vi "Event Handler.vi"(0 "uService Template in":refnum<class "Father of all uServices.lvclass">, 5 "Event type":T1=enum."Message", 7 "Item Name":string, 9 "Data":variant, 11 "error in (no error)":errorcluster) -> (4 "uService Template out":refnum<class "Father of all uServices.lvclass">, 15 "error out":errorcluster)   [LabVIEW 2026, in "TALOS.lvlib" / "Father of all uServices.lvlib" / "Father of all uServices.lvclass"]
uses:
  Father of all uServices.lvclass
  Event Handler Items.ctl
  Father of all uServices.lvclass/Father of all uServices.ctl
  Ancestor/Ancestor/Ancestor.lvclass/Ancestor.ctl
  Classes/Log/Log.lvclass/Log.ctl
  <vilib>/AdvancedString/1D String Array to Delimited String (string).vi
  Support VIs/Generate Error.vi
  Classes/Log/Write.vi
  FGV/Error Memory/Get Error Description.vi
  Support VIs/Get PC name.vi
  Ancestor/Ancestor/Read ID.vi
  Support VIs/Get Class Name.vi
  Support VIs/Date n Time.vi
  FGV/Error Memory/Error Memory Core.vi
  <vilib>/AdvancedString/Delimited String to 1D String Array.vi
  <vilib>/AdvancedString/Delimited String to 1D String Array (string).vi
  Support VIs/Circus Root Path.vi
  FGV/Error Memory/Error Crt Lvl checker.vi
  FGV/Error Memory/Error Memory Core.vi/40c8088d-b597-4017-91af-faa98e00292e.vi
  FGV/Error Memory/Error Memory Core.vi/d4a3ab98-063c-4e44-b43d-fbdcfe6c2be2.vi
  Support VIs/Global Memory.vi
  <vilib>/Utility/LVClass/Get LV Class Name.vi
  Support VIs/Is in Packed Library.vi
  Support VIs/TALOS Root path.vi
  Support VIs/Read CSV worksheet.vi
  Support VIs/Global Constants.vi
  <vilib>/Utility/error.llb/General Error Handler.vi
  <vilib>/Utility/config.llb/Open Config Data.vi
  <vilib>/Utility/config.llb/Get Section Names.vi
  <vilib>/Utility/config.llb/Get Key Names.vi
  <vilib>/Utility/config.llb/Read Key.vi
  <vilib>/Utility/config.llb/Read Key (String).vi
  <vilib>/Utility/config.llb/Close Config Data.vi
  Classes/Log/Rotate.vi
  Ancestor/Ancestor/Ancestor.lvclass
  <vilib>/Comparison/Equal/Equal Functor/Equal Functor.lvclass
  TALOS.lvlib
  Classes/Log/Log.lvclass
panel:
  # "NEVER REGENERATE THE AF MESSAGE!\nIT IS MANUALLY MODIFIED"
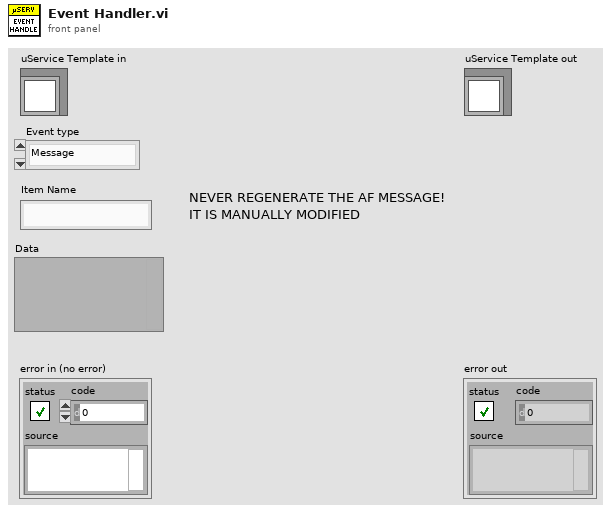
[diagram p1: front panel]
types:
  T1 = typedef "TALOS.lvlib/Father of all uServices.lvlib/Father of all uServices.lvclass/Event Handler Items.ctl" = enum16{"Button Pressed", "Message", "Ready to launch?", "Safe Mode", "Start RUN", "Stop RUN"}
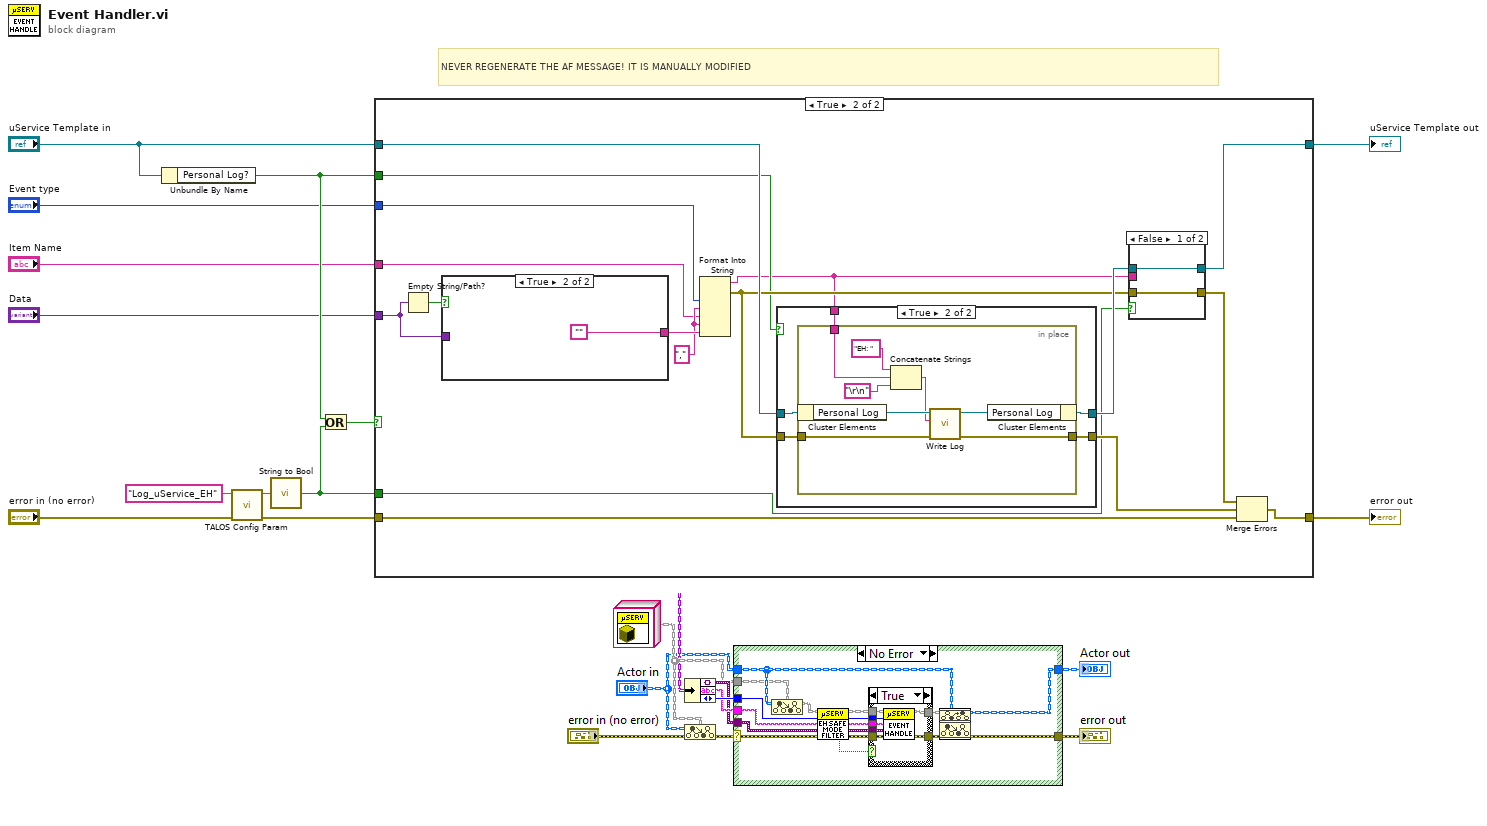
[diagram p0: block diagram]
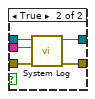
[diagram p3: hidden frame]
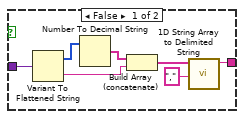
[diagram p4: hidden frame]
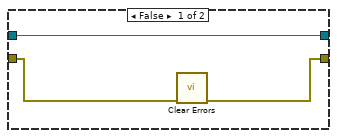
[diagram p5: hidden frame]
diagram:
  # "NEVER REGENERATE THE AF MESSAGE! IT IS MANUALLY MODIFIED"
  n1 = Unbundle By Name("uService Template in") -> ("Personal Log?"=w6:bool)
  n2 = call "TALOS Config Param.vi"("error in (no error)"="error in (no error)", "Parameter Name"="Log_uService_EH") -> ("error out"=w9:errorcluster, "Output"=w11:string)  [unwired: 8 in]
  n3 = call "String to Bool.vi"("String"=w11) -> ("Boolean"=w5:bool)
  n4 = Or(x=w6, y=w5) -> (x .or. y?=w7:bool)
  n5 = case shown="True" w7 {
    tunnel: [w14 w32] -> w13
    tunnel: [w15 w29] -> w12
    tunnel: "Item Name" -> [_ w27]
    tunnel: "Event type" -> [_ w26]
    tunnel: "uService Template in" -> [w14 w22]
    tunnel: "Data" -> [_ w25]
    tunnel: w9 -> [w15 w24]
    tunnel: w6 -> [_ w18]
    tunnel: w5 -> [_ w16]
    frame False {
    }
    frame True {
      w28 = "," ("input 2")
      n6 = Empty String/Path?(string/path=w25) -> (empty?=w31:bool)
      n7 = case shown="True" w31 {
        tunnel: w25 -> [w46 _]
        tunnel: [w40 "" ("Empty String Constant")] -> w30
        frame False {
          n8 = Variant To Flattened String(Variant=w46) -> (data string=w42:string, 1:w45:i16[])
          n9 = Number To Decimal String(number=w45) -> (decimal integer string=w43:string[])  [unwired: 1 in]
          n10 = Build Array (concatenate)(w43, w42) -> (w41:string[])
          n11 = call-poly <vilib>:"1D String Array to Delimited String.vi"("delimiter"=",", "string array"=w41) -> ("delimited string"=w40:string)  [unwired: 9 in]
        }
        frame True {
        }
      }
      n12 = Format Into String(w26, w28, w27, w28, w30) -> (resulting string=w17:string, error out=w19:errorcluster)  [unwired: 3 in]
      n13 = case shown="True" w18 {
        tunnel: [w48 w55] -> w23
        tunnel: w22 -> [w48 w54]
        tunnel: [w49 w53] -> w20
        tunnel: w19 -> [w50 w52]
        tunnel: w17 -> [_ w51]
        frame False {
          n14 = call <vilib>:"Clear Errors.vi"("error in (no error)"=w50) -> ("error out"=w49:errorcluster)  [unwired: 5 in, 1 out]
        }
        frame True {
          n15 = in-place {
            in-place-border: [w61] -> w53
            in-place-border: w52 -> [w60]
            in-place-border: w51 -> [w59]
            n16 = in-place-cluster #1(w54) -> ("Personal Log"=w63:refnum<class "Log.lvclass">)
            n17 = Concatenate Strings("EH: " ("string"), w59, "\r\n") -> (w58:string)
            n18 = call "Write Log.vi"("error in (no error)"=w60, "Text"=w58, "Log in"=w63) -> ("error out"=w61:errorcluster, "Log out"=w62:refnum<class "Log.lvclass">)  [unwired: 7 in]
            n19 = in-place-cluster #1("Personal Log"=w62) -> (w55:refnum<class "Father of all uServices.lvclass">)
          }
        }
      }
      n20 = case shown="False" w16 {
        tunnel: [w34 w39] -> w32
        tunnel: w23 -> [w34 w38]
        tunnel: [w33 w37] -> w21
        tunnel: w19 -> [w33 w36]
        tunnel: w17 -> [_ w35]
        frame False {
        }
        frame True {
          n21 = call "System Log.vi"("error in (no error)"=w36, "Text to log"=w35, "uService Template in"=w38) -> ("error out"=w37:errorcluster, "uService Template out"=w39:refnum<class "Father of all uServices.lvclass">)  [unwired: 7 in]
        }
      }
      n22 = Merge Errors(w21, w20, w24) -> (w29:errorcluster)
    }
  }
  "error out" <- w12
  "uService Template out" <- w13
